vi "日志报警状态存储 (子VI).vi"() -> ()   [LabVIEW 2016, in "斯坦道CODMn.lvlib"]
uses:
  <vilib>/ptbypt/NI_PtbyPt.lvlib
panel:
  out "多列列表框":i32(listbox)
  out "CODMn工作状态":T1(ring)
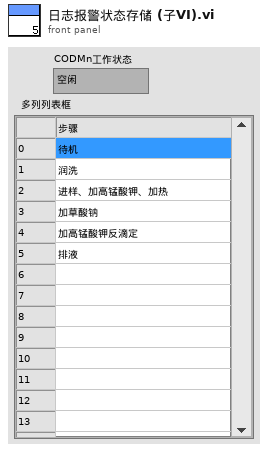
[diagram p1: front panel]
types:
  T1 = enum16{"空闲", "水样测试", "标样核查", "零点核查", "跨度核查", "空白测试", "平行样测试", "质控样", "空白校准", "标样校准", "加标回收"}
  T2 = cluster{"时间标识":timestamp, "设备":string, "日志信息":string}
  T3 = cluster{"时间标识":timestamp, "参数":string, "日志信息":string, "流程参数":string}
  T4 = cluster{"ORP故障":bool, "温控器故障":bool, "加热故障":bool, "高锰酸钾报警":bool, "草酸钠报警":bool, "测量错误":bool, "校零错误":bool, "校标错误":bool, " 进水样超量程":bool, "排液阀故障":bool, "60分钟超时报警":bool, "进样无液体报警":bool}
  T5 = cluster{"时间标识":timestamp, "设备":string, "日志信息":string, "流程参数":string}
  T6 = cluster{"测量量程":dbl, "测量精度":dbl, "测量间隔":dbl, "消解温度":dbl, "消解时长":dbl, "空白校准时间":timestamp, "曲线截距":dbl, "曲线斜率":dbl, "测量检出限":dbl, "测量信号值":dbl, "线性相关系数":dbl, "二次多项式系数":dbl, "标样校准时间":timestamp, "稀释倍数":dbl, "三项式系数":dbl, "空白标定系数":dbl, "量程系数":dbl, "F0/ORPA":dbl, "F1/ORPB":dbl, "F2/ORPK":dbl, "F3":dbl, "F4":dbl, "F5":dbl, "F6":dbl, "F7":dbl, "X0/滴定数":dbl, "量程":dbl}
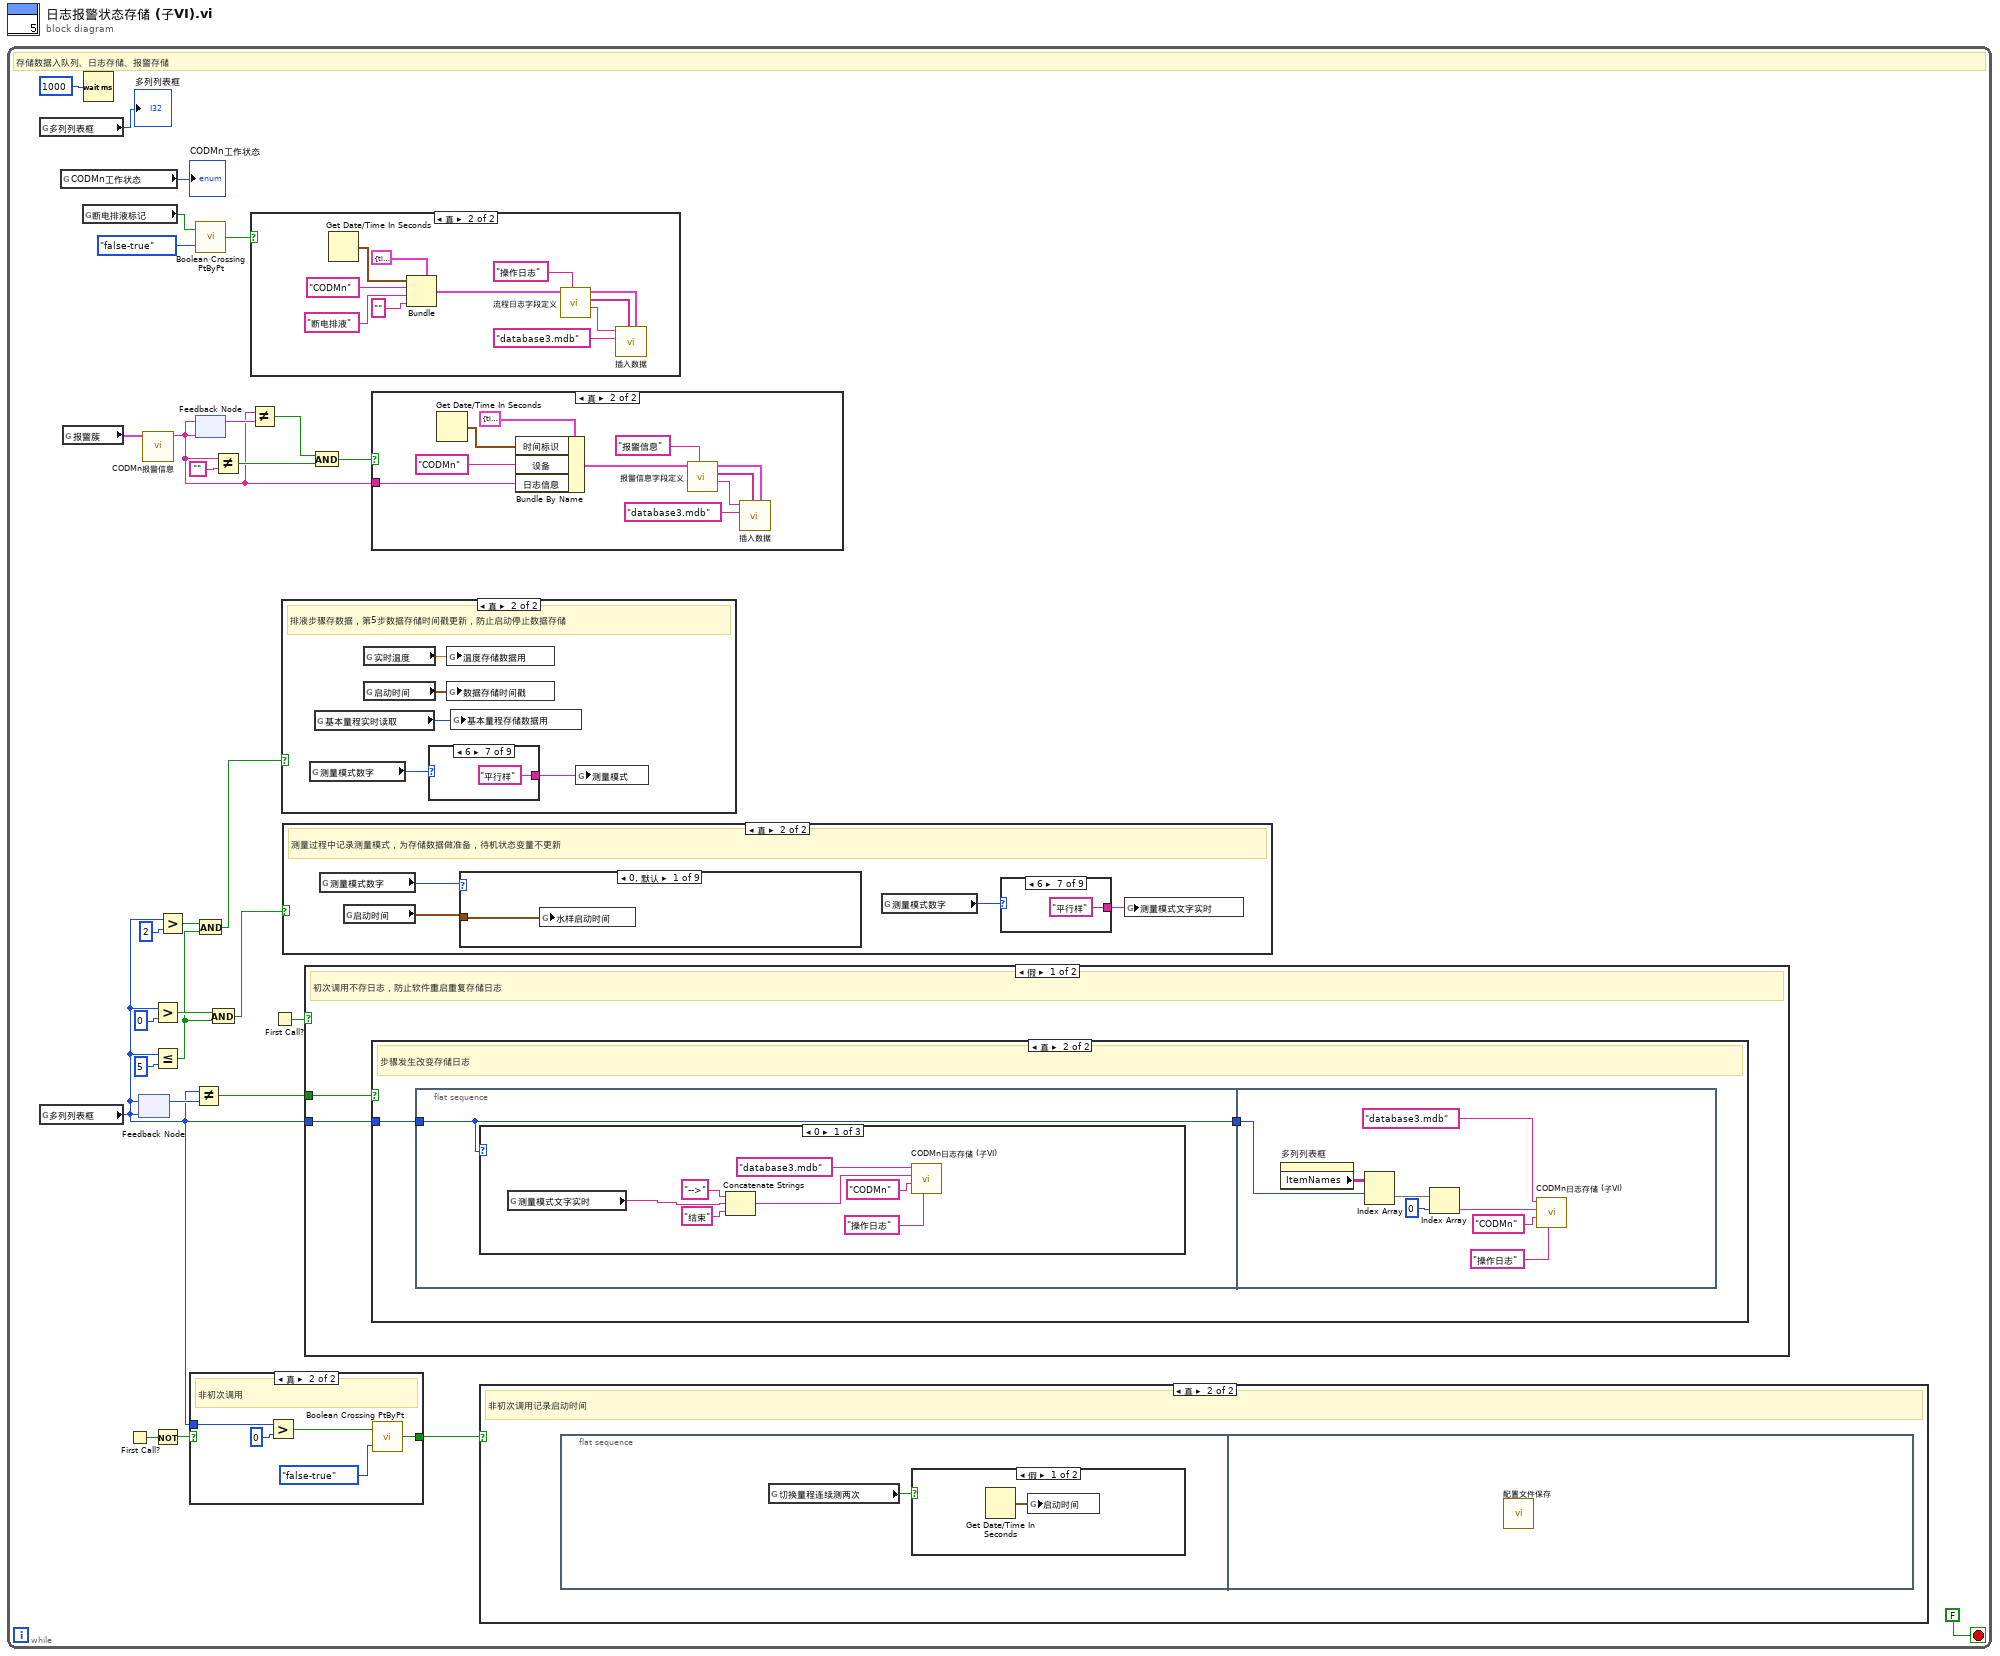
[diagram p0: block diagram]
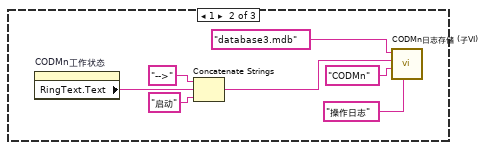
[diagram p3: hidden frame]
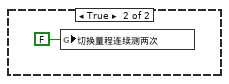
[diagram p10: hidden frame]
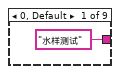
[diagram p12: hidden frame]
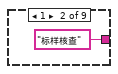
[diagram p13: hidden frame]
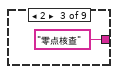
[diagram p14: hidden frame]
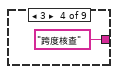
[diagram p15: hidden frame]
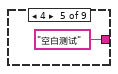
[diagram p16: hidden frame]
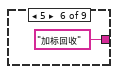
[diagram p17: hidden frame]
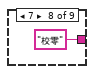
[diagram p18: hidden frame]
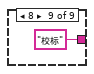
[diagram p19: hidden frame]
diagram:
  n1 = while {
    stop <- FALSE stop-if-true
    # "存储数据入队列、日志存储、报警存储"
    n2 = global read "运行时序全局变量.vi" "多列列表框"() -> (→"多列列表框":i32)
    n3 = global read "运行时序全局变量.vi" "多列列表框"() -> (w3:i32)
    n4 = global read "COD测量模式全局.vi" "CODMn工作状态"() -> (→"CODMn工作状态":T1)
    n5 = global read "COD内部交互全局.vi" "报警簇"() -> (w10:T4)
    n6 = global read "COD内部交互全局.vi" "断电排液标记"() -> (w9:bool)
    n7 = Wait (ms)(milliseconds to wait=u32 1000 ("等待时间（毫秒）")) -> ()  [unwired: 1 out]
    n8 = First Call?() -> (First Call?: T/F=w13:bool)
    n9 = feedback #1(w3) -> (w24:i32)
    n10 = feedback-in #1(w3) -> ()
    n11 = call "CODMn报警信息.vi"("报警簇"=w10) -> ("CODMN报警信息"=w14:string)  [unwired: 10 in]
    n12 = Greater?(x=w3, y=u16 0) -> (0:w29:bool)
    n13 = Less Or Equal?(x=w3, y=u16 5) -> (x <= y?=w4:bool)
    n14 = Not(x=w13) -> (.not. x?=w11:bool)
    n15 = Greater?(x=w3, y=u16 2) -> (0:w5:bool)
    n16 = case shown="真" w11 {
      selector: w11 -> [w57 _]
      tunnel: w3 -> [_ w59]
      tunnel: [w57 w58] -> w12
      frame False {
      }
      frame True {
        # "非初次调用"
        n17 = Greater?(x=w59, y=u16 0) -> (0:w62:bool)
        n18 = call <vilib>:"Boolean Crossing PtByPt.vi"("direction"=enum16{"either", "false-true", "true-false"}."false-true", "input"=w62) -> ("crossing"=w58:bool)  [unwired: 1 in]
      }
    }
    n19 = Not Equal?(x=w3, y=w24) -> (x != y?=w25:bool)
    n20 = call <vilib>:"Boolean Crossing PtByPt.vi"("direction"=enum16{"either", "false-true", "true-false"}."false-true", "input"=w9) -> ("crossing"=w20:bool)  [unwired: 1 in]
    n21 = feedback #2(w14) -> (w15:string)
    n22 = feedback-in #2(w14) -> ()
    n23 = And(x=w5, y=w4) -> (x .and. y?=w2:bool)
    n24 = And(x=w29, y=w4) -> (x .and. y?=w1:bool)
    n25 = Not Equal?(x=w14, y="") -> (x != y?=w19:bool)
    n26 = Not Equal?(x=w14, y=w15) -> (x != y?=w16:bool)
    n27 = case shown="真" w20 {
      frame False {
      }
      frame True {
        n28 = Get Date/Time In Seconds() -> (seconds since 1Jan1904=w78:timestamp)
        n29 = Bundle(cluster=T3 {"时间标识"=timestamp(0 s since 1904-01-01), "参数"="", "日志信息"="", "流程参数"=""} ("data in"), "时间标识"=w78, "参数"="CODMn" ("table输入"), "日志信息"="断电排液", "流程参数"="" ("table输入")) -> (w76:T3)
        n30 = call "流程日志字段定义.vi"("table输入"="操作日志", "data in"=w76) -> ("table输出"=w81:string, "columns"=w82:string[], "data out"=w83:T5)  [unwired: 7 in]
        n31 = call "插入数据.vi"("data"=w83, "columns"=w82, "database"="database3.mdb", "table"=w81) -> ()  [unwired: 7 in, 1 out]
      }
    }
    n32 = First Call?() -> (First Call?: T/F=w26:bool)
    n33 = case shown="真" w2 {
      frame False {
      }
      frame True {
        # "排液步骤存数据，第5步数据存储时间戳更新，防止启动停止数据存储"
        n34 = global read "COD内部交互全局.vi" "测量模式数字"() -> (w108:i32)
        n35 = global read "COD内部交互全局.vi" "基本量程实时读取"() -> (w110:enum16{"L", "H", "AUTO"})
        n36 = global read "COD内部交互全局.vi" "实时温度"() -> (w111:dbl)
        n37 = global read "CODMn断电保存全局变量.vi" "启动时间"() -> (w112:timestamp)
        n38 = case shown="6" w108 {
          tunnel: ["水样测试" ("测量模式") "标样核查" ("测量模式") "零点核查" ("测量模式") "跨度核查" ("测量模式") "空白测试" ("测量模式") "加标回收" ("测量模式") "平行样" ("测量模式") "校零" ("测量模式") "校标" ("测量模式")] -> w109
          frame 0, Default {
          }
          frame 1 {
          }
          frame 2 {
          }
          frame 3 {
          }
          frame 4 {
          }
          frame 5 {
          }
          frame 6 {
          }
          frame 7 {
          }
          frame 8 {
          }
        }
        n39 = global write "COD内部交互全局.vi" "温度存储数据用"(w111) -> ()
        n40 = global write "COD内部交互全局.vi" "数据存储时间戳"(w112) -> ()
        n41 = global write "COD内部交互全局.vi" "基本量程存储数据用"(w110) -> ()
        n42 = global write "COD测量模式全局.vi" "测量模式"(w109) -> ()
      }
    }
    n43 = case shown="真" w1 {
      frame False {
      }
      frame True {
        # "测量过程中记录测量模式，为存储数据做准备，待机状态变量不更新"
        n44 = global read "COD内部交互全局.vi" "测量模式数字"() -> (w89:i32)
        n45 = global read "CODMn断电保存全局变量.vi" "启动时间"() -> (w90:timestamp)
        n46 = case shown="0, 默认" w89 {
          tunnel: w90 -> [w100 _ _ _ _ w101 _ w102 w105]
          frame 0, Default {
            n47 = global write "COD测量模式全局.vi" "水样启动时间"(w100) -> ()
          }
          frame 1 {
          }
          frame 2 {
          }
          frame 3 {
          }
          frame 4 {
          }
          frame 5 {
            n48 = global write "COD测量模式全局.vi" "加标回收启动时间"(w101) -> ()
          }
          frame 6 {
          }
          frame 7 {
            n49 = global read "CODMn断电保存全局变量.vi" "CODMn仪器参数"() -> (w104:T6)
            n50 = Bundle By Name(cluster=w104, "空白校准时间"=w102) -> (w103:T6)
            n51 = global write "CODMn断电保存全局变量.vi" "CODMn仪器参数"(w103) -> ()
          }
          frame 8 {
            n52 = global read "CODMn断电保存全局变量.vi" "CODMn仪器参数"() -> (w107:T6)
            n53 = Bundle By Name(cluster=w107, "标样校准时间"=w105) -> (w106:T6)
            n54 = global write "CODMn断电保存全局变量.vi" "CODMn仪器参数"(w106) -> ()
          }
        }
        n55 = global read "COD内部交互全局.vi" "测量模式数字"() -> (w87:i32)
        n56 = case shown="6" w87 {
          tunnel: ["水样测试" ("测量模式") "标样核查" ("测量模式") "零点核查" ("测量模式") "跨度核查" ("测量模式") "空白测试" ("测量模式") "加标回收" ("测量模式") "平行样" ("测量模式") "校零" ("测量模式") "校标" ("测量模式")] -> w88
          frame 0, Default {
          }
          frame 1 {
          }
          frame 2 {
          }
          frame 3 {
          }
          frame 4 {
          }
          frame 5 {
          }
          frame 6 {
          }
          frame 7 {
          }
          frame 8 {
          }
        }
        n57 = global write "COD测量模式全局.vi" "测量模式文字实时"(w88) -> ()
      }
    }
    n58 = case shown="假" w26 {
      tunnel: w25 -> [w31 _]
      tunnel: w3 -> [w30 _]
      frame False {
        # "初次调用不存日志，防止软件重启重复存储日志"
        n59 = case shown="真" w31 {
          tunnel: w30 -> [_ w33]
          frame False {
          }
          frame True {
            # "步骤发生改变存储日志"
            n60 = flat-sequence {
              tunnel: w33 -> [w34]
              tunnel: [w34] -> w32
              tunnel: w32 -> [w54]
              frame #0 {
                n61 = case shown="0" w34 {
                  frame 0 {
                    n62 = global read "COD测量模式全局.vi" "测量模式文字实时"() -> (w35:string)
                    n63 = Concatenate Strings("-->", w35, "结束" ("字符串")) -> (w41:string)
                    n64 = call "CODMn日志存储 (子VI).vi"("table输入"="操作日志", "参数"="CODMn" ("table输入"), "日志信息"=w41, "database"="database3.mdb") -> ()  [unwired: 8 in]
                  }
                  frame 1 {
                    n65 = property on="CODMn工作状态" class="Enum (严格)"() -> ("RingText.Text"=w42:string)  [unwired: 2 in, 2 out]
                    n66 = Concatenate Strings("-->", w42, "启动" ("字符串")) -> (w43:string)
                    n67 = call "CODMn日志存储 (子VI).vi"("table输入"="操作日志", "参数"="CODMn" ("table输入"), "日志信息"=w43, "database"="database3.mdb") -> ()  [unwired: 8 in]
                  }
                  frame 2, Default {
                  }
                }
              }
              frame #1 {
                n68 = property on="多列列表框" class="MCListbox (严格)"() -> ("ItemNames"=w49:string[][])  [unwired: 2 in, 2 out]
                n69 = Index Array(array=w49, index (row)=w54) -> (element=w52:string[])  [unwired: 1 in]
                n70 = Index Array(array=w52, index=0 ("索引")) -> (element=w50:string)
                n71 = call "CODMn日志存储 (子VI).vi"("table输入"="操作日志", "参数"="CODMn" ("table输入"), "日志信息"=w50, "database"="database3.mdb") -> ()  [unwired: 8 in]
              }
            }
          }
        }
      }
      frame True {
      }
    }
    n72 = And(x=w16, y=w19) -> (x .and. y?=w17:bool)
    n73 = case shown="真" w17 {
      tunnel: w14 -> [_ w63]
      frame False {
      }
      frame True {
        n74 = Get Date/Time In Seconds() -> (seconds since 1Jan1904=w65:timestamp)
        n75 = Bundle By Name(cluster=T2 {"时间标识"=timestamp(0 s since 1904-01-01), "设备"="", "日志信息"=""} ("data in"), "时间标识"=w65, "设备"="CODMn", "日志信息"=w63) -> (w66:T2)
        n76 = call "报警信息字段定义.vi"("table输入"="报警信息", "data in"=w66) -> ("table输出"=w70:string, "columns"=w71:string[], "data out"=w72:T2)  [unwired: 7 in]
        n77 = call "插入数据.vi"("data"=w72, "columns"=w71, "database"="database3.mdb", "table"=w70) -> ()  [unwired: 7 in, 1 out]
      }
    }
    n78 = case shown="真" w12 {
      frame False {
      }
      frame True {
        # "非初次调用记录启动时间"
        n79 = flat-sequence {
          frame #0 {
            n80 = global read "COD内部交互全局.vi" "切换量程连续测两次"() -> (w84:bool)
            n81 = case shown="假" w84 {
              frame False {
                n82 = Get Date/Time In Seconds() -> (seconds since 1Jan1904=w85:timestamp)
                n83 = global write "CODMn断电保存全局变量.vi" "启动时间"(w85) -> ()
              }
              frame True {
                n84 = global write "COD内部交互全局.vi" "切换量程连续测两次"(FALSE ("切换量程连续测两次")) -> ()
              }
            }
          }
          frame #1 {
            n85 = call "配置文件保存.vi"() -> ()  [unwired: 12 in]
          }
        }
      }
    }
  }
